vi "Destroy.vi"(8 "error in (no error)":errorcluster, 11 "reference in":refnum<class "ImageFacialDetection.lvclass">) -> (0 "error out":errorcluster, 3 "reference out":refnum<class "ImageFacialDetection.lvclass">)   [LabVIEW 2017, in "ImageFacialDetection.lvclass"]
uses:
  ImageFacialDetection.lvclass
  <vilib>/Enthought/Python Integration Toolkit/Python Integration Toolkit.lvlib
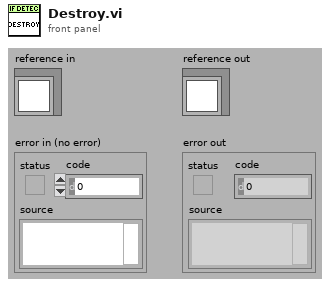
[diagram p1: front panel]
types:
  T1 = typedef "ImageFacialDetection.lvclass/ObjectAttributes.ctl" = cluster{"Path to Python Module (.py File)":path, "Python Session ID":T2}
  T2 = typedef "Python Integration Toolkit.lvlib/Session ID.ctl" = u64
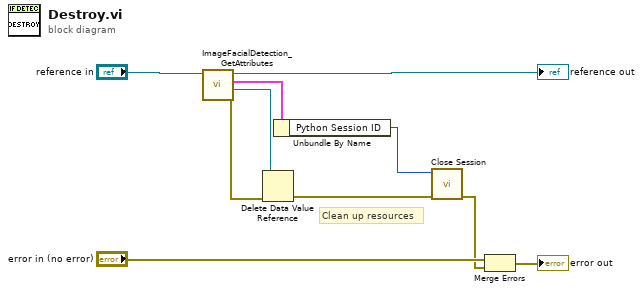
[diagram p0: block diagram]
diagram:
  # "Clean up resources"
  n1 = call "ImageFacialDetection_GetAttributes.vi"("reference in"="reference in") -> ("error out"=w7:errorcluster, "DataRef"=w6:refnum<data-value>, "Data"=w5:T1, "reference out"=→"reference out":refnum<class "ImageFacialDetection.lvclass">)  [unwired: 7 in]
  n2 = Delete Data Value Reference(data value reference=w6, error in=w7) -> (error out=w2:errorcluster)  [unwired: 1 out]
  n3 = Unbundle By Name(w5) -> ("Python Session ID"=w3:T2)
  n4 = call <vilib>:"Close Session.vi"("error in (no error)"=w2, "Session ID"=w3) -> ("error out"=w1:errorcluster)  [unwired: 9 in]
  n5 = Merge Errors("error in (no error)", w1) -> (→"error out":errorcluster)
